vi "File Range.vi"(8 "error in (no error)":errorcluster, 9 "End(%)":dbl, 10 "start(%)":dbl, 11 "Data Loader in":refnum<class "Data Loader.lvclass">) -> (0 "error out":errorcluster, 3 "Data Loader out":refnum<class "Data Loader.lvclass">)   [LabVIEW 2020, in "Data Loader.lvlib" / "Data Loader.lvclass"]
uses:
  Data Loader.lvclass
  Data Loader.lvclass/Data Loader.ctl
  Data Types/Abstrut Data/Abstruct Data Type.lvclass/Abstruct Data Type.ctl
  MVVM Framework/MVVM Abstruct Model/MVVM Abstruct Model/MVVM Abstruct Model.lvclass/MVVM Abstruct Model.ctl
  Views/Data Interface/Data Interface Messages/Update Data Msg/Update Data Msg.lvclass/Update Data Msg.ctl
  <vilib>/ActorFramework/Message Enqueuer/Message Enqueuer.lvclass/Message Enqueuer.ctl
  Data Types/Abstrut Data/Accessors/Read Length.vi
  Data Types/Abstrut Data/Accessors/Write Index.vi
  Data Types/Abstrut Data/Accessors/Write Range.vi
  MVVM Framework/MVVM Abstruct Model/MVVM Abstruct Model/Accessor/Read ActorMap-Views.vi
  Accessor/Read Data File.lvclass.vi
  Data Types/Abstrut Data/Accessors/Read Selected Channels.vi
  <vilib>/ActorFramework/Message Enqueuer/Enqueue.vi
  Views/Data Interface/Data Interface Messages/Update Data Msg/Update Data Msg.lvclass
  C:/Program Files (x86)/National Instruments/LabVIEW 2020/vi.lib/ActorFramework/Message/Message.lvclass
  <vilib>/ActorFramework/Message Priority Queue/Priority Enqueue.vi
  <vilib>/ActorFramework/Message Enqueuer/Message Enqueuer.lvclass
  Depden On/ActorMap/ActorMap.lvclass
  Data Types/Abstrut Data/Abstruct Data Type.lvclass
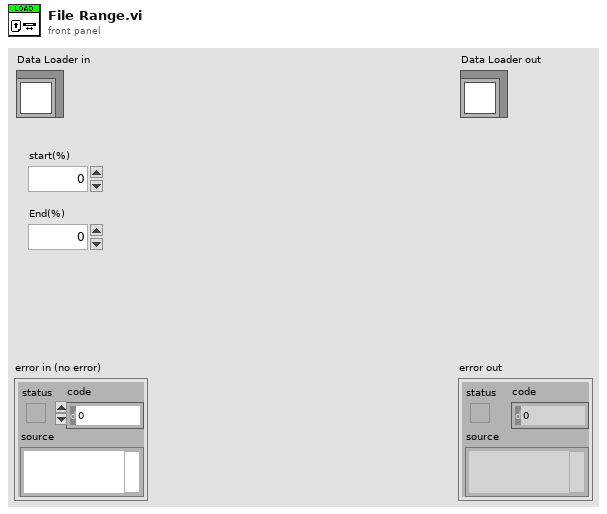
[diagram p1: front panel]
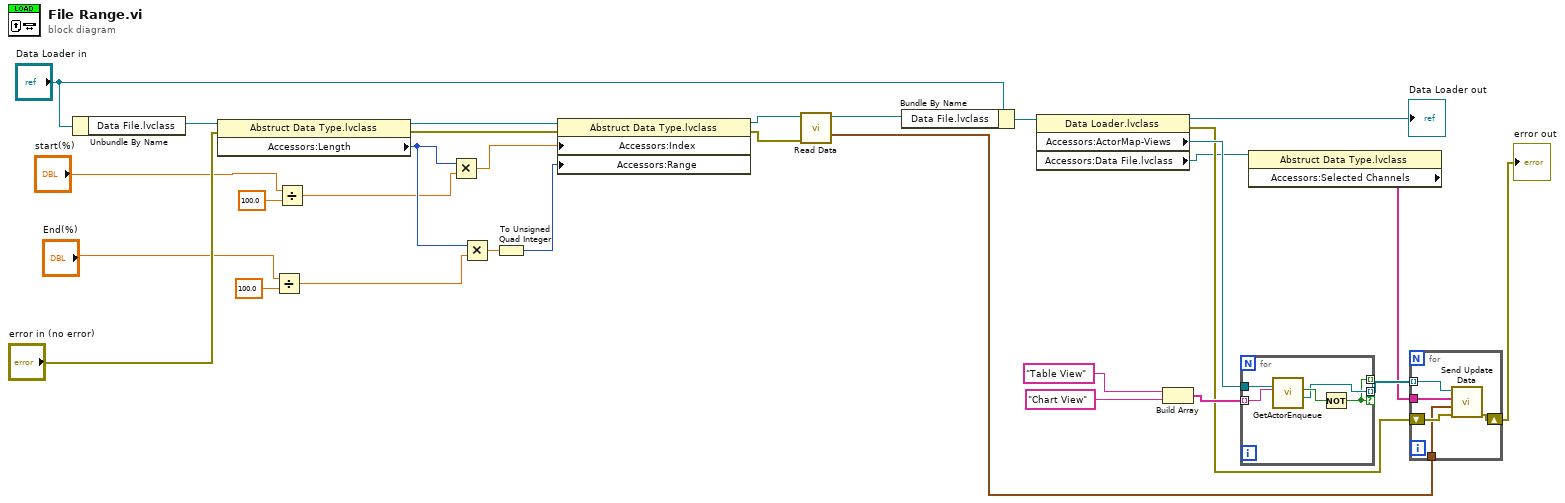
[diagram p0: block diagram]
diagram:
  n1 = Unbundle By Name("Data Loader in") -> ("Data File.lvclass"=w30:refnum<class "Abstruct Data Type.lvclass">)
  n2 = property class="Abstruct Data Type.lvclass"(reference=w30, error in="error in (no error)") -> (reference out=w28:refnum<class "Abstruct Data Type.lvclass">, error out=w25:errorcluster, "Accessors:Length"=w29:u64)
  n3 = Divide(x="End(%)", y=100.0) -> (x/y=w4:dbl)
  n4 = Divide(x="start(%)", y=100.0) -> (x/y=w6:dbl)
  n5 = Multiply(x=w29, y=w6) -> (x*y=w26:dbl)
  n6 = Multiply(x=w29, y=w4) -> (x*y=w2:dbl)
  n7 = To Unsigned Quad Integer(1:w2) -> (0:w1:u64)
  n8 = property class="Abstruct Data Type.lvclass"(reference=w28, error in=w25, "Accessors:Index"=w26, "Accessors:Range"=w1) -> (reference out=w23:refnum<class "Abstruct Data Type.lvclass">, error out=w21:errorcluster)
  n9 = call-dynamic "Read Data.vi"("error in (no error)"=w21, "Abstruct Data Type in"=w23) -> ("data"=w13:waveform(dbl)[], "Abstruct Data Type out"=w22:refnum<class "Abstruct Data Type.lvclass">)  [unwired: 7 in, 1 out]
  n10 = Bundle By Name(cluster="Data Loader in", "Data File.lvclass"=w22) -> (w14:refnum<class "Data Loader.lvclass">)
  n11 = property class="Data Loader.lvclass"(reference=w14) -> (reference out=→"Data Loader out":refnum<class "Data Loader.lvclass">, error out=w15:errorcluster, "Accessors:ActorMap-Views"=w20:refnum<class "ActorMap.lvclass">, "Accessors:Data File.lvclass"=w11:refnum<class "Abstruct Data Type.lvclass">)  [unwired: 1 in]
  n12 = Build Array("Table View", "Chart View") -> (w18:string[])
  n13 = for {
    tunnel: w20 -> [w35]
    tunnel: w18 -> [w34] mode=indexing
    tunnel: [w31] -> _ mode=indexing
    tunnel: [w32] -> w16 mode=indexing if=w31
    n14 = call "GetActorEnqueue.vi"("name"=w34, "ActorMap in"=w35) -> ("Enqueue"=w32:refnum<class "Message Enqueuer.lvclass">, "key not found?"=w33:bool)  [unwired: 6 in, 2 out]
    n15 = Not(x=w33) -> (.not. x?=w31:bool)
  }
  n16 = property class="Abstruct Data Type.lvclass"(reference=w11) -> ("Accessors:Selected Channels"=w10:string[])  [unwired: 1 in, 2 out]
  n17 = for {
    tunnel: w16 -> [w40] mode=indexing
    shift-right: [w38] -> w9
    shift-left: w15 -> [w39]
    tunnel: w13 -> [w37]
    tunnel: w10 -> [w36]
    n18 = call "Send Update Data.vi"("error in (no error)"=w39, "data"=w37, "Channel Names"=w36, "Message Enqueuer"=w40) -> ("error out"=w38:errorcluster)  [unwired: 6 in, 1 out]
  }
  "error out" <- w9
